vi "createInstance.vi"(8 "error in (no error)":errorcluster, 9 "salTypedefPath":path=path "C:/LSSTSW/SAL_LabVIEW_Interface/SALTypedefs/Control 2.ctl", 10 "instanceDirectory":path, 11 "OpenConnectionInstance in":refnum<class "OpenConnectionInstance.lvclass">) -> (0 "error out":errorcluster, 3 "OpenConnectionInstance out":refnum<class "OpenConnectionInstance.lvclass">)   [LabVIEW 2012, in "OpenConnectionInstance.lvclass"]
uses:
  OpenConnectionInstance.lvclass
  PolymorphicInstance/PolymorphicInstance.lvclass
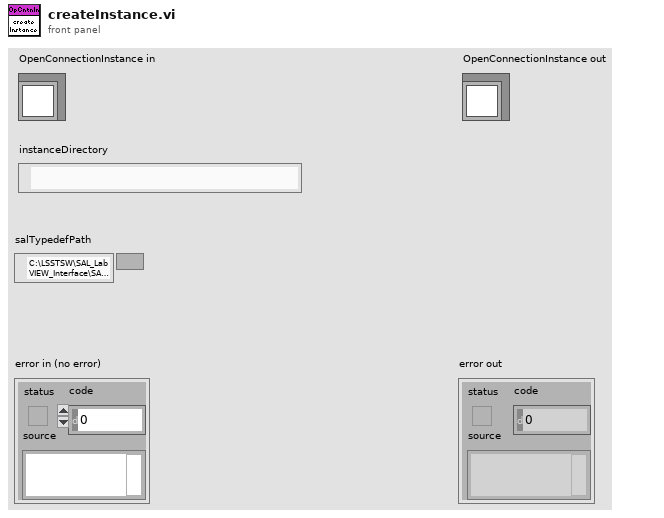
[diagram p1: front panel]
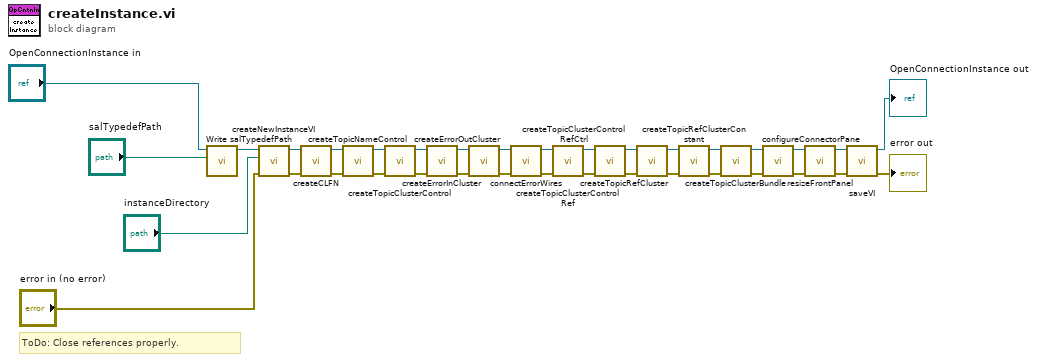
[diagram p0: block diagram]
diagram:
  # "ToDo: Close references properly."
  n1 = call "Write salTypedefPath.vi"("salTypedefPath"="salTypedefPath", "PolymorphicInstance in"="OpenConnectionInstance in") -> ("PolymorphicInstance out"=w29:refnum<class "OpenConnectionInstance.lvclass">)  [unwired: 9 in]
  n2 = call "createNewInstanceVI.vi"("error in (no error)"="error in (no error)", "instanceDirectory"="instanceDirectory", "PolymorphicInstance in"=w29) -> ("error out"=w35:errorcluster, "PolymorphicInstance out"=w34:refnum<class "OpenConnectionInstance.lvclass">)  [unwired: 7 in]
  n3 = call "createCLFN.vi"("error in (no error)"=w35, "PolymorphicInstance in"=w34) -> ("error out"=w31:errorcluster, "PolymorphicInstance out"=w32:refnum<class "OpenConnectionInstance.lvclass">)  [unwired: 8 in]
  n4 = call "createTopicNameControl.vi"("error in (no error)"=w31, "OpenConnectionInstance in"=w32) -> ("error out"=w26:errorcluster, "OpenConnectionInstance out"=w27:refnum<class "OpenConnectionInstance.lvclass">)  [unwired: 8 in]
  n5 = call "createTopicClusterControl.vi"("error in (no error)"=w26, "PolymorphicInstance in"=w27) -> ("error out"=w24:errorcluster, "PolymorphicInstance out"=w25:refnum<class "OpenConnectionInstance.lvclass">)  [unwired: 8 in]
  n6 = call "createErrorInCluster.vi"("error in (no error)"=w24, "PolymorphicInstance in"=w25) -> ("error out"=w22:errorcluster, "PolymorphicInstance out"=w23:refnum<class "OpenConnectionInstance.lvclass">)  [unwired: 8 in]
  n7 = call "createErrorOutCluster.vi"("error in (no error)"=w22, "PolymorphicInstance in"=w23) -> ("error out"=w20:errorcluster, "PolymorphicInstance out"=w21:refnum<class "OpenConnectionInstance.lvclass">)  [unwired: 8 in]
  n8 = call "connectErrorWires.vi"("error in (no error)"=w20, "PolymorphicInstance in"=w21) -> ("error out"=w18:errorcluster, "PolymorphicInstance out"=w19:refnum<class "OpenConnectionInstance.lvclass">)  [unwired: 8 in]
  n9 = call "createTopicClusterControlRef.vi"("error in (no error)"=w18, "PolymorphicInstance in"=w19) -> ("error out"=w16:errorcluster, "PolymorphicInstance out"=w17:refnum<class "OpenConnectionInstance.lvclass">)  [unwired: 8 in]
  n10 = call "createTopicClusterControlRefCtrl.vi"("error in (no error)"=w16, "PolymorphicInstance in"=w17) -> ("error out"=w14:errorcluster, "PolymorphicInstance out"=w15:refnum<class "OpenConnectionInstance.lvclass">)  [unwired: 8 in]
  n11 = call "createTopicRefCluster.vi"("error in (no error)"=w14, "PolymorphicInstance in"=w15) -> ("error out"=w12:errorcluster, "PolymorphicInstance out"=w13:refnum<class "OpenConnectionInstance.lvclass">)  [unwired: 8 in]
  n12 = call "createTopicRefClusterConstant.vi"("error in (no error)"=w12, "OpenConnectionInstance in"=w13) -> ("error out"=w10:errorcluster, "OpenConnectionInstance out"=w11:refnum<class "OpenConnectionInstance.lvclass">)  [unwired: 8 in]
  n13 = call "createTopicClusterBundle.vi"("error in (no error)"=w10, "OpenConnectionInstance in"=w11) -> ("error out"=w8:errorcluster, "OpenConnectionInstance out"=w9:refnum<class "OpenConnectionInstance.lvclass">)  [unwired: 8 in]
  n14 = call-dynamic "configureConnectorPane.vi"("error in (no error)"=w8, "OpenConnectionInstance in"=w9) -> ("error out"=w3:errorcluster, "OpenConnectionInstance out"=w5:refnum<class "OpenConnectionInstance.lvclass">)  [unwired: 8 in]
  n15 = call "resizeFrontPanel.vi"("error in (no error)"=w3, "PolymorphicInstance in"=w5) -> ("error out"=w2:errorcluster, "PolymorphicInstance out"=w4:refnum<class "OpenConnectionInstance.lvclass">)  [unwired: 8 in]
  n16 = call "saveVI.vi"("error in (no error)"=w2, "PolymorphicInstance in"=w4) -> ("error out"=→"error out":errorcluster, "PolymorphicInstance out"=→"OpenConnectionInstance out":refnum<class "OpenConnectionInstance.lvclass">)  [unwired: 8 in]
